vi "Plot Helper (Matrix).vi"(4 "Plot ID":i32, 6 "z matrix":sgl[][](array[numeric]), 8 "error in (no error)":errorcluster, 9 "y matrix":sgl[][](array[numeric]), 10 "x matrix":sgl[][](array[numeric]), 11 "3D Plot lvclass Array in":refnum<class "3D Plot Datatype.lvclass">[](array[class])) -> (0 "error out":errorcluster, 3 "3D Plot lvclass Array out":refnum<class "3D Plot Datatype.lvclass">[](array[class]))   [LabVIEW 2020, in "3D Waterfall Datatype.lvclass"]
doc: "Graphs the surface of the data and the area on the y-axis below the data points. Multiple references to this VI generate multiple plots for the same graph."
uses:
  <vilib>/Math Plots/3D Math Plots/3D Waterfall/3D Waterfall Datatype/3D Waterfall Datatype.lvclass
  <vilib>/Math Plots/3D Math Plots/3D Plot/3D Plot Datatype/3D Plot Datatype.lvclass
  e:/builds/penguin/labview/branches/2020/dev/dist/vi.lib/Math Plots/3D Math Plots/3D Plot/3D Plot Datatype/3D Plot Datatype.lvclass
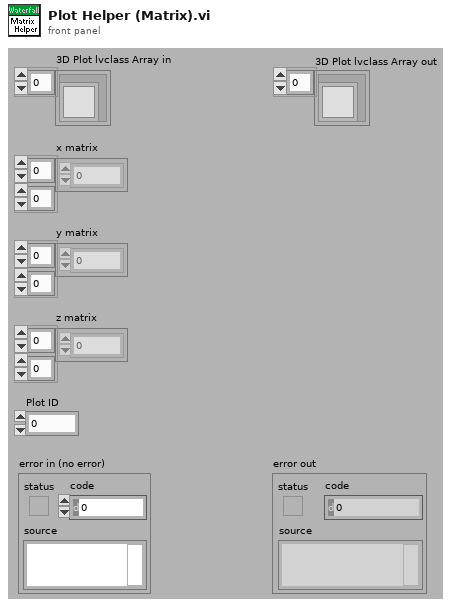
[diagram p1: front panel]
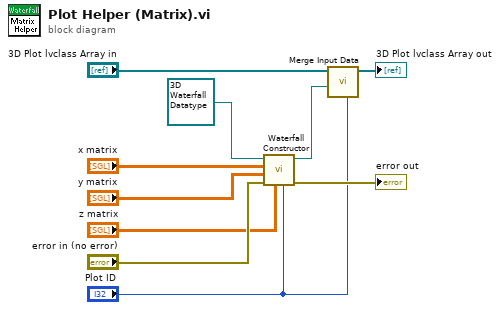
[diagram p0: block diagram]
diagram:
  n1 = call <vilib>:"Waterfall Constructor.vi"("Plot ID"="Plot ID", "z matrix"="z matrix", "error in (no error)"="error in (no error)", "y matrix"="y matrix", "x matrix"="x matrix", "3D Waterfall Datatype.lvclass in"=refnum<class "3D Waterfall Datatype.lvclass"> refnum ("3D Mesh Datatype.lvclass")) -> ("error out"=→"error out":errorcluster, "3D Waterfall Datatype.lvclass out"=w5:refnum<class "3D Waterfall Datatype.lvclass">)  [unwired: 1 in, 3 out]
  n2 = call <vilib>:"Merge Input Data.vi"("Plot ID"="Plot ID", "3D Plot lvclass in"=w5, "3D Plot lvclass Array in"="3D Plot lvclass Array in") -> ("3D Plot lvclass Array out"=→"3D Plot lvclass Array out":refnum<class "3D Plot Datatype.lvclass">[])  [unwired: 8 out]
